vi "Acquisition Message Loop.vi"(8 "error in (no error)":errorcluster, 9 "Data Queue":refnum<queue>, 10 "Data Notifier":refnum<notifier>, 11 "Message Queues":T1) -> (0 "error out":errorcluster)   [LabVIEW 2013, in "Cal Inst Acquisition.lvlib"]
doc: "Message loop for handling messages pertaining to the acquisition of data from the hardware."
uses:
  Cal Inst Acquisition.lvlib
  support/Message Queue/All Message Queues.ctl
  support/Message Queue/Message Cluster.ctl
  controls/electrical2.ctl
  Hardware Configuration.ctl
  Acquisition State.ctl
  support/Message Queue/Enqueue Message (Single).vi
  <vilib>/Utility/error.llb/Error Cluster From Error Code.vi
  <vilib>/ErrorRing/Error Ring.xnode
  support/Message Queue/Cal Inst Message Queue.lvlib
  Libraries/California Instruments iX Series/California Instruments iX Series.lvlib
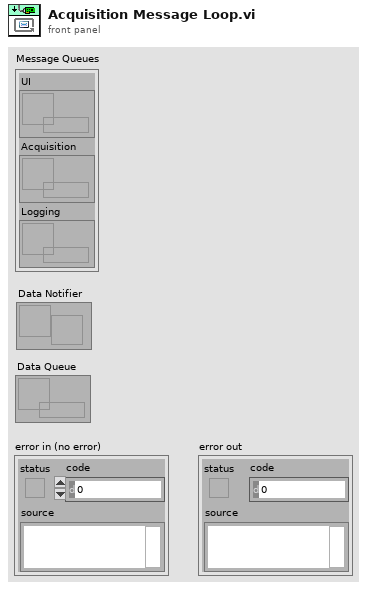
[diagram p1: front panel]
types:
  T1 = typedef "Cal Inst Message Queue.lvlib/All Message Queues.ctl" = cluster{"UI":refnum<queue>, "Acquisition":refnum<queue>, "Logging":refnum<queue>}
  T2 = typedef "Cal Inst Acquisition.lvlib/Hardware Configuration.ctl" = cluster{"VISA Refnum in":refnum<visa-resource-name>, "Serial Configuration":cluster{"Baud Rate":u32, "Flow Control":u16}, "Voltage Level (0V)":dbl}
  T3 = typedef "Cal Inst Acquisition.lvlib/Acquisition State.ctl" = enum16{"Idle", "Acquiring"}
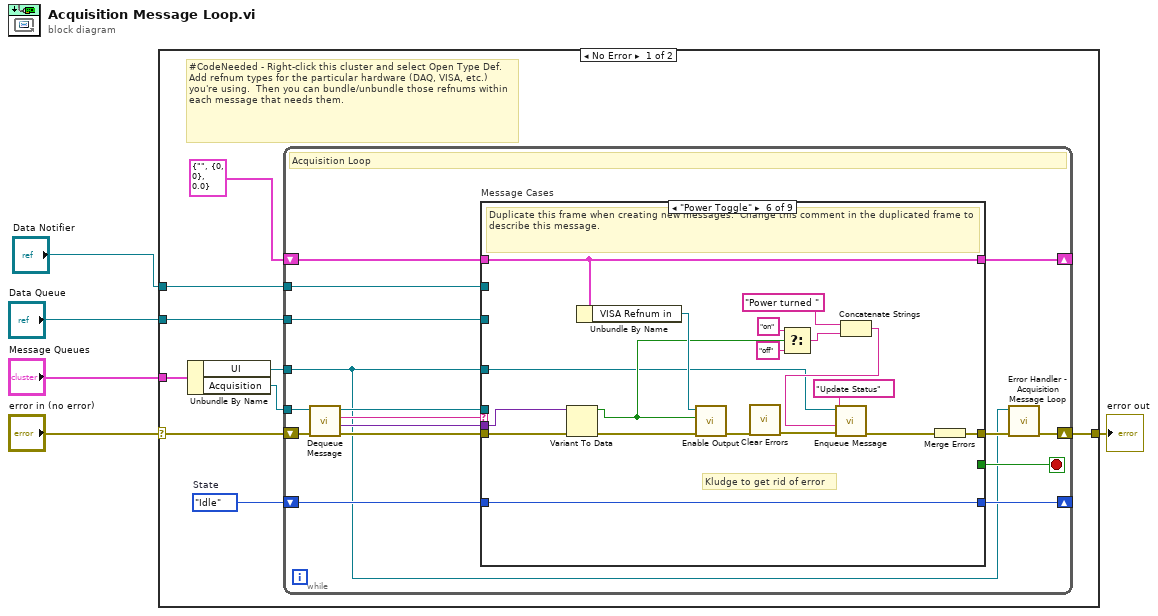
[diagram p0: block diagram]
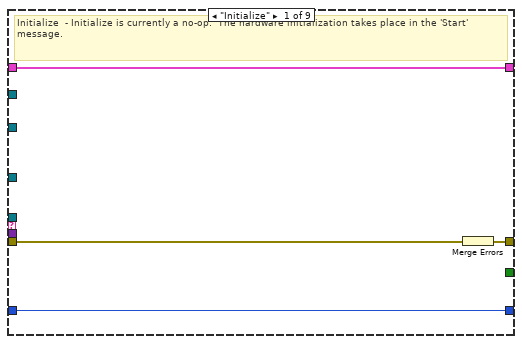
[diagram p2: hidden frame]
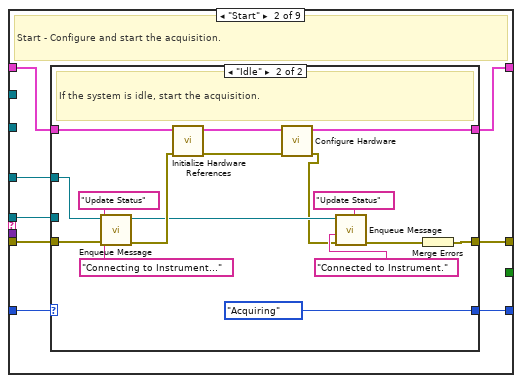
[diagram p3: hidden frame]
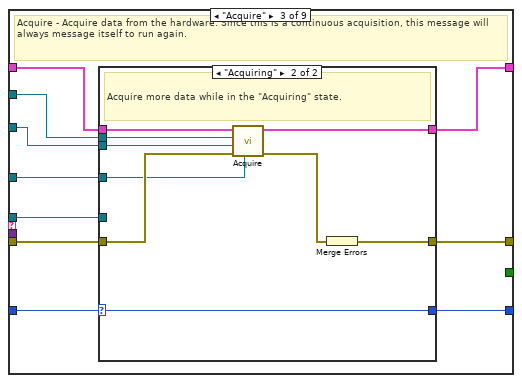
[diagram p5: hidden frame]
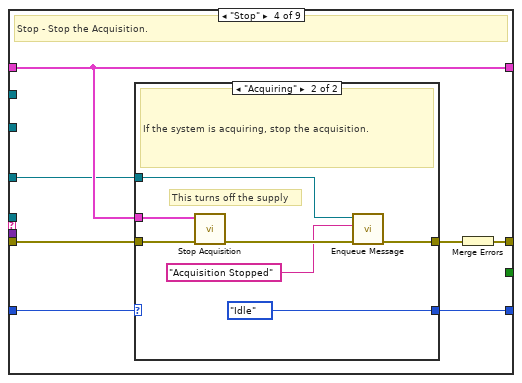
[diagram p7: hidden frame]
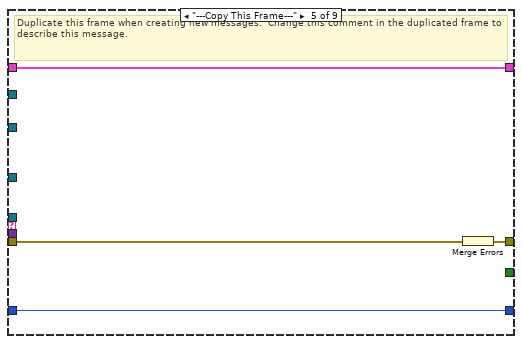
[diagram p9: hidden frame]
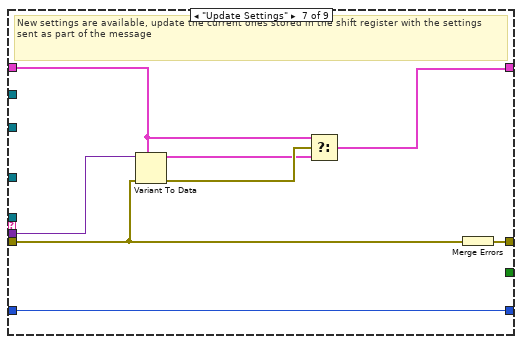
[diagram p10: hidden frame]
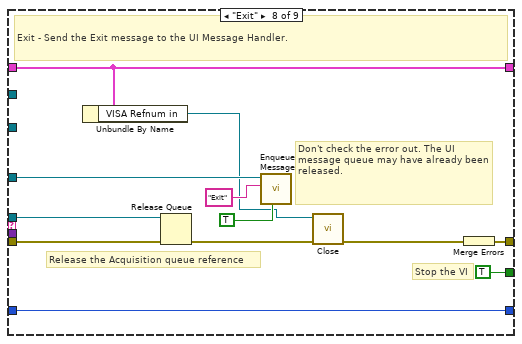
[diagram p11: hidden frame]
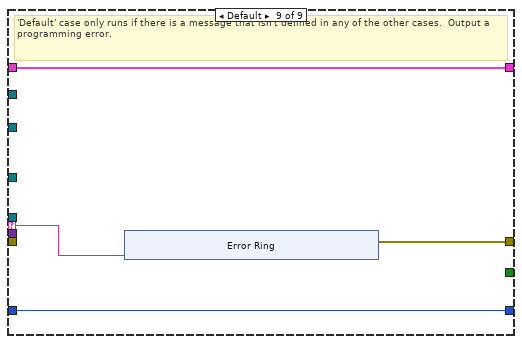
[diagram p12: hidden frame]
diagram:
  n1 = case shown="No Error" "error in (no error)" {
    selector: "error in (no error)" -> [w10 w153]
    tunnel: "Message Queues" -> [w14 _]
    tunnel: [w12 w153] -> w4
    tunnel: "Data Notifier" -> [w8 _]
    tunnel: "Data Queue" -> [w7 _]
    frame No Error {
      w6 = Acquisition_State."Idle"  # State
      # "#CodeNeeded - Right-click this cluster and select Open Type Def.  Add refnum types for the particular hardware (DAQ, VISA, etc.) you're using.  Then you can bundle/unbundle those refnums within each message that needs them."
      n2 = Unbundle By Name(w14) -> ("UI"=w9:refnum<queue>, "Acquisition"=w13:refnum<queue>)
      n3 = while {
        tunnel: w13 -> [w23]
        shift-right: [w29] -> _
        shift-left: T2 {"VISA Refnum in"="", "Serial Configuration"={"Baud Rate"=0, "Flow Control"=0}, "Voltage Level (0V)"=0.0} ("Data Cluster") -> [w30]
        shift-right: [w18] -> w12
        shift-left: w10 -> [w27]
        tunnel: w9 -> [w15]
        tunnel: w8 -> [w22]
        tunnel: w7 -> [w21]
        shift-right: [w19] -> _
        shift-left: w6 -> [w20]
        stop <- w28 stop-if-true
        # "Acquisition Loop"
        n4 = call "Dequeue Message.vi"("error in (no error)"=w27, "Message Queue"=w23) -> ("error out"=w26:errorcluster, "Message Data"=w24:variant, "Message"=w25:string, "dup Message Queue"=w16:refnum<queue>)  [unwired: 6 in]
        n5 = case "Message Cases" shown="\"Power Toggle\"" w25 {
          selector: w25 -> [_ _ _ _ _ _ _ _ w142]
          tunnel: w16 -> [_ w39 w70 _ _ _ _ w135 _]
          tunnel: w26 -> [w33 w40 w69 w89 w103 w117 w123 w138 _]
          tunnel: [w34 w42 w71 w90 w101 w121 w129 w140 w143] -> w17
          tunnel: w30 -> [w32 w41 w67 w87 w102 w119 w125 w133 w145]
          tunnel: [w32 w38 w68 w87 w102 w119 w124 w133 w145] -> w29
          tunnel: [_ _ _ _ _ _ _ TRUE _] -> w28
          tunnel: w24 -> [_ _ _ _ _ w115 w128 _ _]
          tunnel: w15 -> [_ w35 w62 w84 _ w106 _ w139 _]
          tunnel: w22 -> [_ _ w66 _ _ _ _ _ _]
          tunnel: w21 -> [_ _ w65 _ _ _ _ _ _]
          tunnel: w20 -> [w31 w36 w63 w86 w100 w120 w122 w134 w144]
          tunnel: [w31 w37 w64 w85 w100 w120 w122 w134 w144] -> w19
          frame "Initialize" {
            # "Initialize  - Initialize is currently a no-op.  The hardware initialization takes place in the 'Start' message."
            n6 = Merge Errors(w33) -> (w34:errorcluster)
          }
          frame "Start" {
            # "Start - Configure and start the acquisition."
            n7 = case shown="\"Idle\"" w36 {
              selector: w36 -> [w43 _]
              tunnel: [w44 w61] -> w42
              tunnel: w41 -> [w45 w60]
              tunnel: w40 -> [w44 w52]
              tunnel: w39 -> [_ _]
              tunnel: [w45 w57] -> w38
              tunnel: [w43 Acquisition_State."Acquiring" ("Acquisition State")] -> w37
              tunnel: w35 -> [_ w54]
              frame "Acquiring" {
                # "The system is already acquiring. Ignore the \"Start\" message."
              }
              frame "Idle" {
                # "If the system is idle, start the acquisition."
                n8 = call-poly "Enqueue Message.vi"("error in (no error)"=w52, "Message Data"="Connecting to Instrument..." ("Message"), "Message"="Update Status", "Message Queue"=w54) -> ("error out"=w51:errorcluster, "dup Message Queue"=w49:refnum<queue>)  [unwired: 6 in]
                n9 = call "Initialize Hardware References.vi"("error in (no error)"=w51, "Hardware Resources in"=w60) -> ("error out"=w59:errorcluster, "Hardware Resources out"=w58:T2)  [unwired: 8 in]
                n10 = call "Configure Hardware.vi"("error in (no error)"=w59, "Hardware Resources in"=w58) -> ("error out"=w47:errorcluster, "Hardware Resources out"=w57:T2)  [unwired: 8 in]
                n11 = call-poly "Enqueue Message.vi"("error in (no error)"=w47, "Message Data"="Connected to Instrument." ("Message"), "Message"="Update Status", "Message Queue"=w49) -> ("error out"=w46:errorcluster)  [unwired: 6 in, 1 out]
                n12 = Merge Errors(w46) -> (w61:errorcluster)
              }
            }
          }
          frame "Acquire" {
            # "Acquire - Acquire data from the hardware. Since this is a continuous acquisition, this message will always message itself to run again."
            n13 = case shown="\"Acquiring\"" w63 {
              selector: w63 -> [w72 w78]
              tunnel: [w73 w83] -> w71
              tunnel: w70 -> [_ _]
              tunnel: w69 -> [w73 w77]
              tunnel: [w74 w82] -> w68
              tunnel: w67 -> [w74 w81]
              tunnel: w66 -> [_ w80]
              tunnel: w65 -> [_ w79]
              tunnel: [w72 w78] -> w64
              tunnel: w62 -> [_ w76]
              frame "Idle" {
                # "Ignore \"Acquire\" messages when the acquisition is idle."
              }
              frame "Acquiring" {
                # "Acquire more data while in the \"Acquiring\" state."
                n14 = call "Acquire.vi"("UI"=w76, "error in (no error)"=w77, "Data Queue 2"=w79, "Data Notifier"=w80, "Hardware Resources in"=w81) -> ("error out"=w75:errorcluster, "Hardware Resources out"=w82:T2)  [unwired: 5 in]
                n15 = Merge Errors(w75) -> (w83:errorcluster)
              }
            }
          }
          frame "Stop" {
            # "Stop - Stop the Acquisition."
            n16 = case shown="\"Acquiring\"" w86 {
              selector: w86 -> [w91 _]
              tunnel: w89 -> [w92 w99]
              tunnel: [w92 w95] -> w88
              tunnel: w87 -> [_ w97]
              tunnel: [w91 Acquisition_State."Idle" ("State")] -> w85
              tunnel: w84 -> [_ w94]
              frame "Idle" {
                # "The system is already idle. Ignore the \"Stop\" message."
              }
              frame "Acquiring" {
                # "This turns off the supply"
                # "If the system is acquiring, stop the acquisition."
                n17 = call "Stop Acquisition.vi"("error in (no error)"=w99, "Hardware Resources in"=w97) -> ("error out"=w98:errorcluster)  [unwired: 9 in]
                n18 = call-poly "Enqueue Message.vi"("error in (no error)"=w98, "Message"="Acquisition Stopped", "Message Queue"=w94) -> ("error out"=w95:errorcluster)  [unwired: 7 in, 1 out]
              }
            }
            n19 = Merge Errors(w88) -> (w90:errorcluster)
          }
          frame "---Copy This Frame---" {
            # "Duplicate this frame when creating new messages.  Change this comment in the duplicated frame to describe this message."
            n20 = Merge Errors(w103) -> (w101:errorcluster)
          }
          frame "Power Toggle" {
            # "Kludge to get rid of error"
            # "Duplicate this frame when creating new messages.  Change this comment in the duplicated frame to describe this message."
            n21 = Variant To Data(error in=w117, Variant=w115) -> (data=w114:bool, error out=w116:errorcluster)  [unwired: 1 in]
            n22 = Unbundle By Name(w119) -> ("VISA Refnum in"=w118:refnum<visa-resource-name>)
            n23 = call "Enable Output.vi"("error in (no error)"=w116, "Enable Output (T: Enable)"=w114, "VISA resource name"=w118) -> ("error out"=w105:errorcluster)  [unwired: 7 in, 1 out]
            n24 = call <vilib>:"Clear Errors.vi"("error in (no error)"=w105) -> ("error out"=w104:errorcluster)  [unwired: 6 in]
            n25 = Select(t="on", s=w114, f="off") -> (s? t:f=w111:string)
            n26 = Concatenate Strings("Power turned " ("string"), w111) -> (w107:string)
            n27 = call-poly "Enqueue Message.vi"("error in (no error)"=w104, "Message Data"=w107, "Message"="Update Status", "Message Queue"=w106) -> ("error out"=w108:errorcluster)  [unwired: 6 in, 1 out]
            n28 = Merge Errors(w108) -> (w121:errorcluster)
          }
          frame "Update Settings" {
            # "New settings are available, update the current ones stored in the shift register with the settings sent as part of the message"
            n29 = Variant To Data(error in=w123, type=w125, Variant=w128) -> (data=w126:T2, error out=w127:errorcluster)
            n30 = Select(t=w125, s=w127, f=w126) -> (s? t:f=w124:T2)
            n31 = Merge Errors(w123) -> (w129:errorcluster)
          }
          frame "Exit" {
            # "Don't check the error out. The UI message queue may have already been released."
            # "Release the Acquisition queue reference"
            # "Stop the VI"
            # "Exit - Send the Exit message to the UI Message Handler."
            n32 = Unbundle By Name(w133) -> ("VISA Refnum in"=w132:refnum<visa-resource-name>)
            n33 = Release Queue(queue=w135, error in (no error)=w138) -> (error out=w131:errorcluster)  [unwired: 1 in, 2 out]
            n34 = call-poly "Enqueue Message.vi"("Priority Message? (F)"=TRUE, "Message"="Exit", "Message Queue"=w139) -> ()  [unwired: 7 in, 2 out]
            n35 = call "Close.vi"("error in (no error)"=w131, "VISA resource name"=w132) -> ("error out"=w130:errorcluster)  [unwired: 9 in]
            n36 = Merge Errors(w130) -> (w140:errorcluster)
          }
          frame Default {
            # "'Default' case only runs if there is a message that isn't defined in any of the other cases.  Output a programming error."
            n37 = xnode "Error Ring"("parameter 0"=w142) -> ("error out"=w143:errorcluster)
          }
        }
        n38 = call "Error Handler - Acquisition Message Loop.vi"("error in (no error)"=w17, "Message Queue"=w15) -> ("dup error in"=w18:errorcluster)  [unwired: 8 in, 1 out]
      }
    }
    frame Error {
    }
  }
  "error out" <- w4
